vi "Launcher - Debug Server.vi"(6 "Worker Alias":string="Debug Server", 8 "error in":errorcluster, 9 "Initialization Data":T1, 11 "Debug Server in":refnum<class "Debug Server.lvclass">) -> (0 "error out":errorcluster)   [LabVIEW 2017]
doc: "This VI launches the Head Worker of a Workers application."
uses:
  Workers/Debug Server/Initialization Data.ctl
  Workers/Debug Server/Debug Server.lvclass
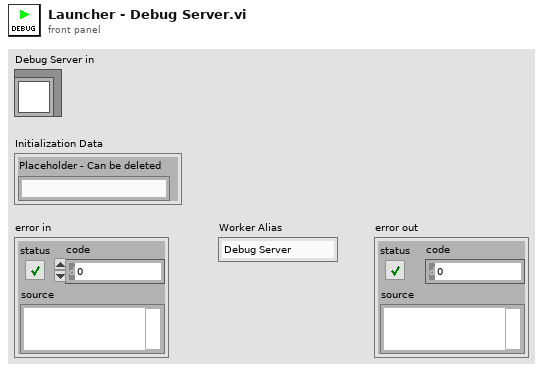
[diagram p1: front panel]
types:
  T1 = typedef "Debug Server.lvclass/Initialization Data.ctl" = cluster{"Placeholder - Can be deleted":string}
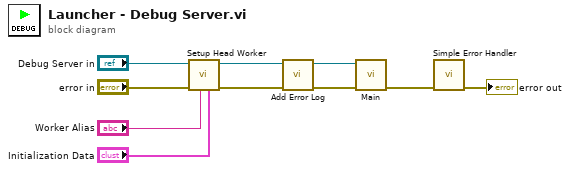
[diagram p0: block diagram]
diagram:
  n1 = call-dynamic "Setup Head Worker.vi"("Initalization Data"="Initialization Data", "Worker Alias"="Worker Alias", "error in"="error in", "Worker_"="Debug Server in") -> ("error out"=w4:errorcluster, "Worker_out"=w5:refnum<class "Debug Server.lvclass">)  [unwired: 6 in]
  n2 = call-dynamic "Add Error Log.vi"("error in"=w4, "Worker"=w5) -> ("error out"=w3:errorcluster, "Worker out"=w2:refnum<class "Debug Server.lvclass">)  [unwired: 8 in]
  n3 = call-dynamic "Main.vi"("error in"=w3, "Debug Server in"=w2) -> ("error out"=w9:errorcluster)  [unwired: 8 in, 1 out]
  n4 = call <vilib>:"Simple Error Handler.vi"("error in (no error)"=w9) -> ("error out"=→"error out":errorcluster)  [unwired: 4 in, 4 out]
